vi "Benchmark - Raster.vi"() -> ()   [LabVIEW 2020, in "Application.lvlib" / "Scene.lvclass"]
uses:
  Scene.lvclass
  3491ce28-564c-437f-89a3-b24602b41f5b.vi
  bff58d7a-0131-44c8-8e39-ec39b410099a.vi
  Benchmark/Benchmark.lvlib
  <vilib>/Analysis/NI_AALBase.lvlib
panel:
  out "Std Dev":dbl format="%.1p"
  out "Mean":dbl format="%.1p"
  out "Histogram Graph":T1(graph)
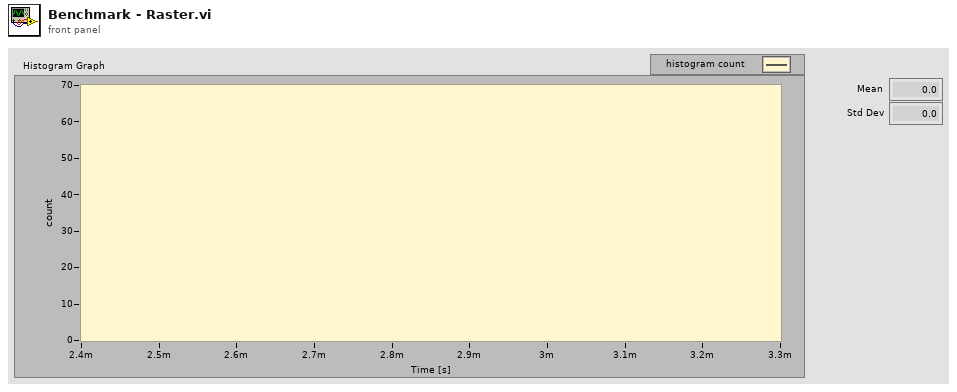
[diagram p1: front panel]
types:
  T1 = cluster{"X Values":dbl[], "Histogram: h(x)":i32[]}
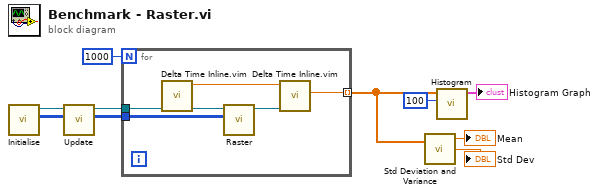
[diagram p0: block diagram]
diagram:
  n1 = call "Initialise.vi"() -> ("Pixel Data out"=w3:u32[][], "Scene out"=w4:refnum<class "Scene.lvclass">)  [unwired: 10 in]
  n2 = call "Update.vi"("Pixel Data in"=w3, "Scene in"=w4) -> ("Pixel Data out"=w1:u32[][], "Scene out"=w2:refnum<class "Scene.lvclass">)  [unwired: 8 in]
  n3 = for {
    N: 1000 -> [_]
    tunnel: [w16] -> w7 mode=indexing
    tunnel: w2 -> [w14]
    tunnel: w1 -> [w11]
    n4 = call "Delta Time Inline.vim"("value in"=w14) -> ("value out"=w13:refnum<class "Scene.lvclass">, "Relative Seconds out [s]"=w15:dbl)  [unwired: 8 in, 1 out]
    n5 = call "Raster.vi"("Pixel Data in"=w11, "Scene in"=w13) -> ("Scene out"=w12:refnum<class "Scene.lvclass">)  [unwired: 8 in, 1 out]
    n6 = call "Delta Time Inline.vim"("value in"=w12, "Relative Seconds in [s]"=w15) -> ("Delta Time [s]"=w16:dbl)  [unwired: 7 in, 2 out]
  }
  n7 = call <vilib>:"Std Deviation and Variance.vi"("X"=w7) -> ("mean"=→"Mean":dbl, "standard deviation"=→"Std Dev":dbl)  [unwired: 1 in, 1 out]
  n8 = call <vilib>:"Histogram.vi"("intervals"=100, "X"=w7) -> ("Histogram Graph"=→"Histogram Graph":T1)  [unwired: 6 in, 3 out]
